vi "TC NI Setup (SubVI).vi"(0 "Refnum in":refnum<k21>, 1 "Refnum out":refnum<k21>, 2 "Min Value (deg C)":dbl, 3 "CJC Value":dbl=25.0 format="%0.2f", 5 "CJC Source":i32(ring)=10116 items=["Built-In"=10200, "Constant Value"=10116, "Channel"=10113], 7 "Max Value (deg C)":dbl=100.0, 9 "Boolean Array In":bool[](array[boolean]), 11 "error in (no error)":errorcluster, 12 "Physical Channels":tag[](array[tag]), 13 "Labels In":string[](array[string]), 14 "Thermocouple Type 1":T1=10073 items=["J"=10072, "K"=10073, "N"=10077, "R"=10082, "S"=10085, "T"=10086, "B"=10047, "E"=10055]) -> (4 "Refnum out":refnum<k21>, 6 "# TC (NI)":i32, 8 "Labels":string[](array[string]), 15 "error out":errorcluster)   [LabVIEW 2011]
uses:
  PAM_Control.ctl
  <vilib>/DAQmx/create/channels.llb/DAQmx Create Channel (AI-Temperature-Thermocouple).vi
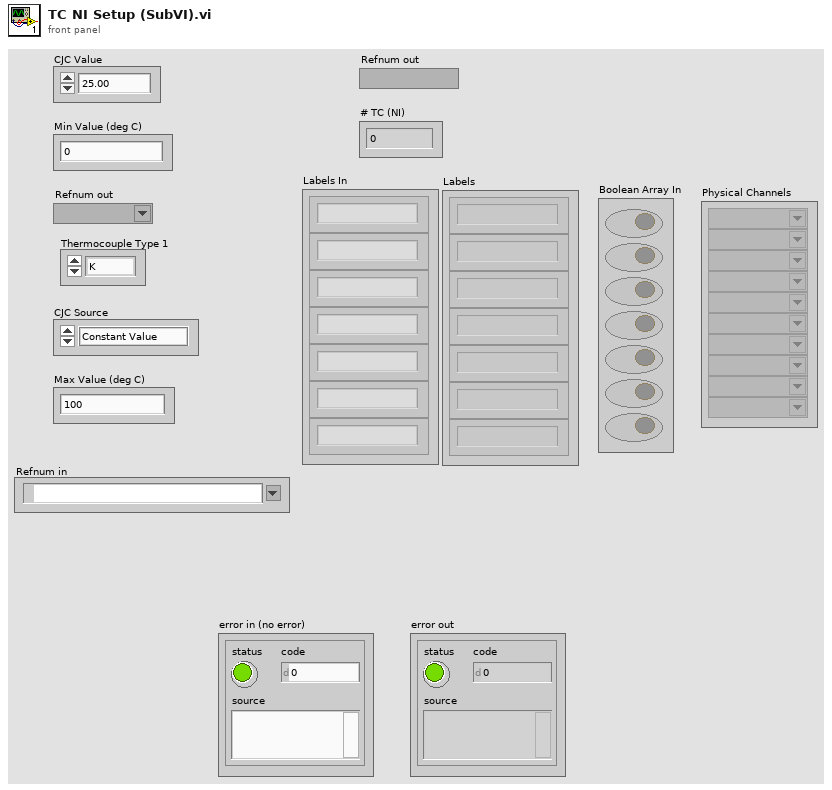
[diagram p1: front panel]
types:
  T1 = typedef "PAM_Control.ctl" = i32
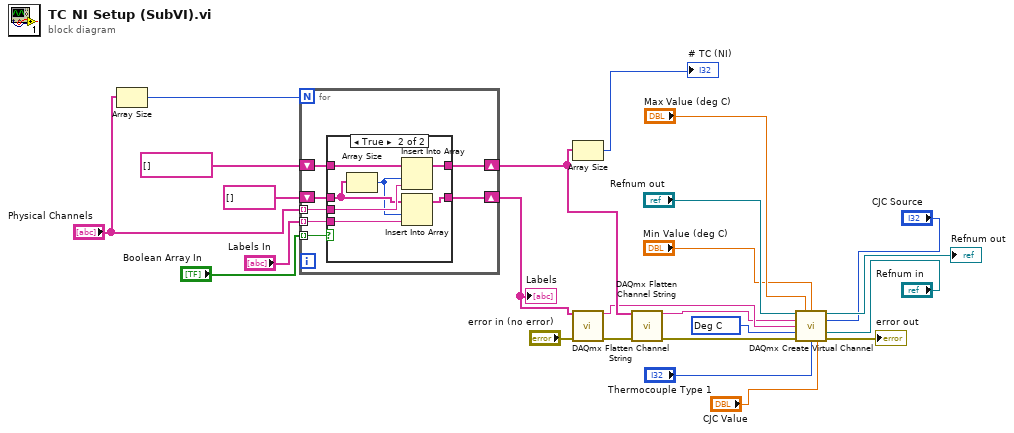
[diagram p0: block diagram]
diagram:
  w10 = 10143 items=["Deg C"=10143, "Deg F"=10144, "Kelvins"=10325, "Deg R"=10145, "From Custom Scale"=10065] ("T Units")
  n1 = Array Size(array="Physical Channels") -> (size(s)=w20:i32)
  n2 = for {
    N: w20 -> [_]
    tunnel: "Physical Channels" -> [w30] mode=indexing
    tunnel: "Labels In" -> [w29] mode=indexing
    tunnel: "Boolean Array In" -> [w31] mode=indexing
    shift-right: [w28] -> w19
    shift-left: tag[] [] -> [w25]
    shift-right: [w27] -> w18
    shift-left: string[] [] -> [w26]
    n3 = case shown="True" w31 {
      tunnel: w30 -> [_ w39]
      tunnel: w29 -> [_ w40]
      tunnel: [w32 w38] -> w28
      tunnel: [w33 w37] -> w27
      tunnel: w26 -> [w33 w35]
      tunnel: w25 -> [w32 w36]
      frame False {
      }
      frame True {
        n4 = Array Size(array=w35) -> (size(s)=w34:i32)
        n5 = Insert Into Array(array=w36, index=w34, new element=w39) -> (w38:tag[])
        n6 = Insert Into Array(array=w35, index=w34, new element=w40) -> (w37:string[])
      }
    }
  }
  "Labels" <- w18
  n7 = Array Size(array=w19) -> (size(s)=→"# TC (NI)":i32)
  n8 = call <vilib>:"DAQmx Flatten Channel String.vi"("names in"=w18, "error in"="error in (no error)") -> ("names out"=w7:string, "error out"=w24:errorcluster)  [unwired: 12 in]
  n9 = call <vilib>:"DAQmx Flatten Channel String.vi"("names in"=w19, "error in"=w24) -> ("names out"=w6:string, "error out"=w9:errorcluster)  [unwired: 12 in]
  n10 = call-poly <vilib>:"DAQmx Create Virtual Channel.vi"("task in"="Refnum out", "maximum value"="Max Value (deg C)", "minimum value"="Min Value (deg C)", "physical channels"=w6, "cjc source"="CJC Source", "name to assign"=w7, "units"=w10, "cjc channel"="Refnum in", "error in"=w9, "thermocouple type"="Thermocouple Type 1", "cjc value"="CJC Value") -> ("task out"=→"Refnum out":refnum<k21>, "error out"=→"error out":errorcluster)  [unwired: 3 in]
